vi "PDC Freq Channels.vi"(7 "Channel Number (1)":i16=1, 8 "error in (no error)":errorcluster {"code" format="%.0x"}, 9 "Channel Band (0:800MHZ BASE)":u16(ring) items=["800MHZ BASE", "800MHZ MOBILE", "1500MHZ BASE", "1500MHZ MOBILE"], 10 "Freq Channels (F:OFF)":bool, 11 "VISA Resource Name":refnum<visa-resource-name>) -> (0 "error out":errorcluster {"code" format="%.0x"}, 3 "VISA Resource Name Out":refnum<visa-resource-name>)   [LabVIEW 2012, in "Agilent ESG Series.lvlib"]
doc: "This VI is used to configure the \"Freq Channels\" parameters."
uses:
  <instrlib>/Agilent ESG Series/Agilent ESG Series.lvlib
panel:
  # "ON"
  # "OFF"
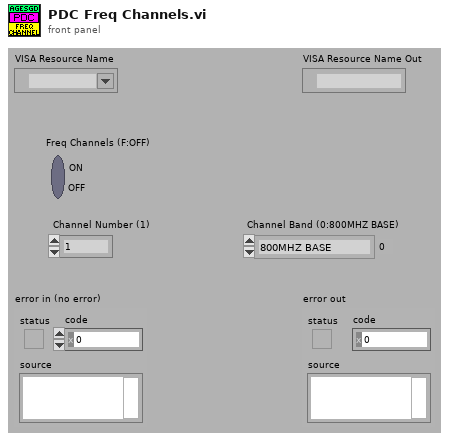
[diagram p1: front panel]
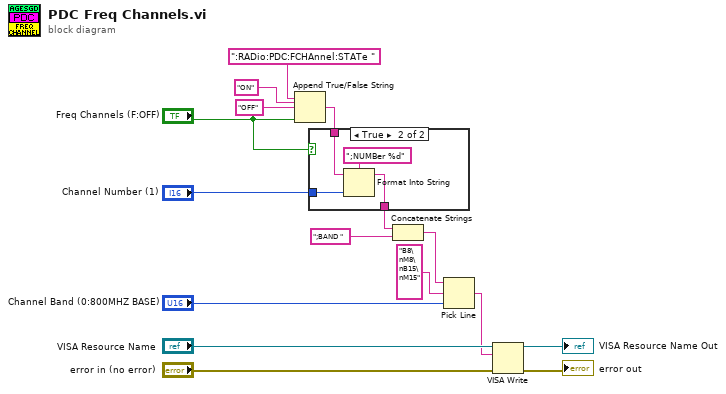
[diagram p0: block diagram]
diagram:
  n1 = Append True/False String(1:"Freq Channels (F:OFF)", 2:"OFF" ("false string"), 3:"ON" ("true string"), 4:":RADio:PDC:FCHAnnel:STATe ") -> (0:w10:string)
  n2 = case shown="True" "Freq Channels (F:OFF)" {
    tunnel: [w17 w20] -> w6
    tunnel: w10 -> [w17 w19]
    tunnel: "Channel Number (1)" -> [_ w18]
    frame False {
    }
    frame True {
      n3 = Format Into String(format string=";NUMBer %d", initial string=w19, w18) -> (resulting string=w20:string)  [unwired: 1 in, 1 out]
    }
  }
  n4 = Concatenate Strings(w6, ";BAND ") -> (w7:string)
  n5 = Pick Line(string ("")=w7, multi-line string="B8\nM8\nB15\nM15" ("true string"), line index="Channel Band (0:800MHZ BASE)") -> (output string=w4:string)
  n6 = VISA Write(VISA resource name="VISA Resource Name", write buffer=w4, error in (no error)="error in (no error)") -> (VISA resource name out=→"VISA Resource Name Out":refnum<visa-resource-name>, error out=→"error out":errorcluster)  [unwired: 1 out]
